vi "Acquire fr Multiple Cameras.vi"() -> (0 "error out":errorcluster)   [LabVIEW 2022 SP3]
uses:
  Anemometry Sub Vis/Globals/Meas_global.vi
  Camera Server/Globals/CamServer global.vi
panel:
  out "element":path
  out "Name 4":string
  out "Image 4":T1(plugin-control)
  out "Name 3":string
  out "Image 3":T1(plugin-control)
  out "Name 2":string
  out "Image 2":T1(plugin-control)
  out "Name 1":string
  out "Image 1":T1(plugin-control)
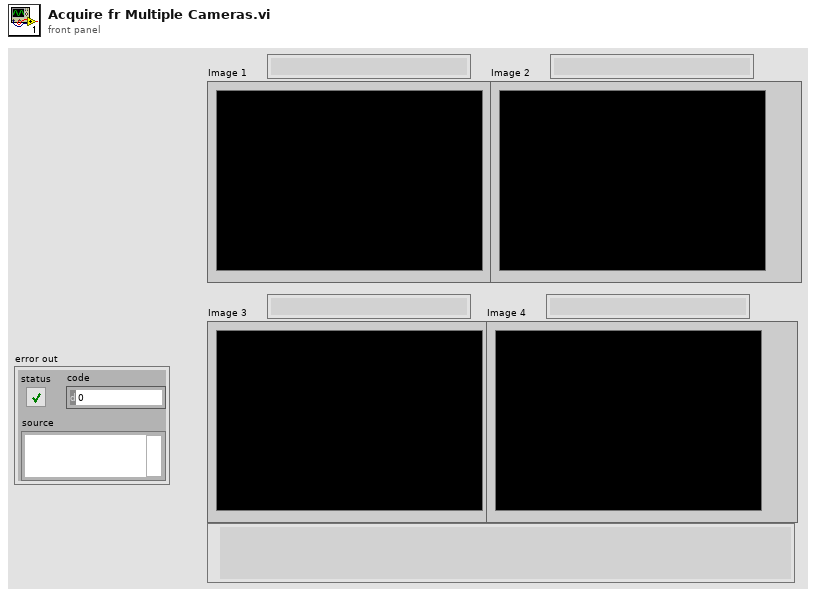
[diagram p1: front panel]
types:
  T1 = typedef "IMAQ Image.ctl" = refnum<image>
  T2 = typedef "Camera enum.ctl" = string
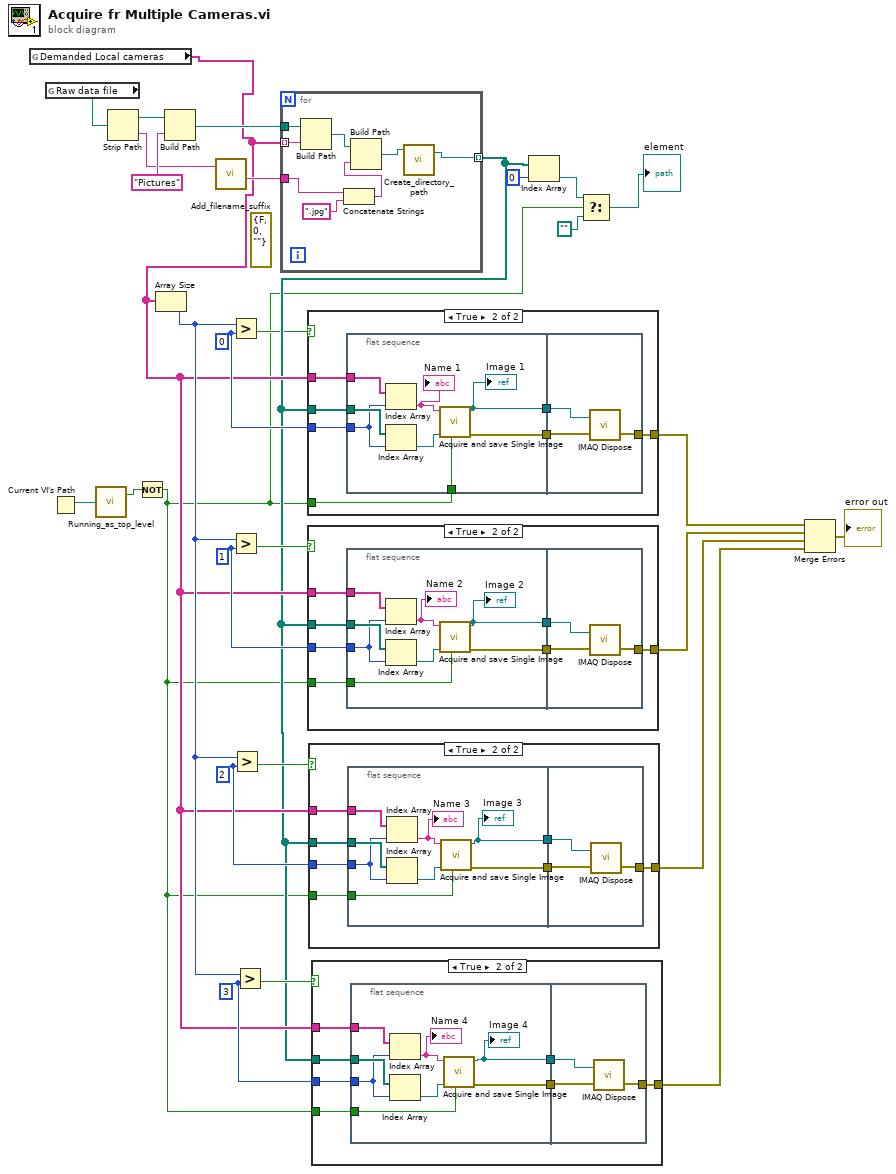
[diagram p0: block diagram]
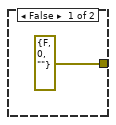
[diagram p2: hidden frame]
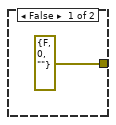
[diagram p3: hidden frame]
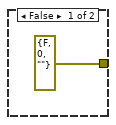
[diagram p4: hidden frame]
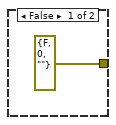
[diagram p5: hidden frame]
diagram:
  w14 = 3 ("y")
  w15 = 2 ("y")
  w16 = 1 ("y")
  w17 = 0 ("y")
  (unwired) errorcluster {"status"=FALSE, "code"=0, "source"=""} ("error IO")
  n1 = global read "CamServer global.vi" "Demanded Local cameras"() -> (w10:T2[])
  n2 = global read "Meas_global.vi" "Raw data file"() -> (w25:path)
  n3 = Current VI's Path() -> (path=w9:path)
  n4 = call "Running_as_top_level.vi"("Vi path name"=w9) -> ("Top Level"=w8:bool)  [unwired: 1 out]
  n5 = Strip Path(path=w25) -> (stripped path=w27:path, name=w24:string)
  n6 = Not(x=w8) -> (.not. x?=w1:bool)
  n7 = Array Size(array=w10) -> (size(s)=w18:i32)
  n8 = Build Path(base path=w27, name or relative path="Pictures") -> (appended path=w28:path)
  n9 = call "Add_filename_suffix.vi"("Filename"=w24) -> ("Base name"=w29:string)  [unwired: 1 in, 3 out]
  n10 = Greater?(x=w18, y=w17) -> (0:w5:bool)
  n11 = Greater?(x=w18, y=w16) -> (0:w21:bool)
  n12 = Greater?(x=w18, y=w15) -> (0:w20:bool)
  n13 = Greater?(x=w18, y=w14) -> (0:w19:bool)
  n14 = for {
    tunnel: w28 -> [w37]
    tunnel: w10 -> [w32] mode=indexing
    tunnel: w29 -> [w33]
    tunnel: [w30] -> w7 mode=indexing
    n15 = Build Path(base path=w37, name or relative path=w32) -> (appended path=w36:path)
    n16 = Concatenate Strings(w33, ".jpg" ("string")) -> (w34:string)
    n17 = Build Path(base path=w36, name or relative path=w34) -> (appended path=w31:path)
    n18 = call "Create_directory_path.vi"("Path name"=w31) -> ("Path name Out"=w30:path)  [unwired: 2 in, 1 out]
  }
  n19 = case shown="True" w5 {
    tunnel: w10 -> [_ w45]
    tunnel: w7 -> [_ w44]
    tunnel: [errorcluster {"status"=FALSE, "code"=0, "source"=""} ("error out") w43] -> w23
    tunnel: w17 -> [_ w40]
    tunnel: w1 -> [_ w39]
    frame False {
    }
    frame True {
      n20 = flat-sequence {
        tunnel: w45 -> [w53]
        tunnel: w44 -> [w52]
        tunnel: [w50] -> w42
        tunnel: [w49] -> w41
        tunnel: w40 -> [w48]
        tunnel: w39 -> [w46]
        tunnel: [w55] -> w43
        tunnel: w42 -> [w56]
        tunnel: w41 -> [w54]
        frame #0 {
          n21 = Index Array(array=w53, index=w48) -> (element=w47:T2)
          "Name 1" <- w47
          n22 = Index Array(array=w52, index=w48) -> (element=w51:path)
          n23 = call "Acquire and save Single Image.vi"("Save image?"=w46, "File Path"=w51, "Camera Name"=w47) -> ("error out"=w50:errorcluster, "Image"=w49:T1)  [unwired: 4 in]
          "Image 1" <- w49
        }
        frame #1 {
          n24 = call "IMAQ Dispose"("Image"=w54, "error in (no error)"=w56) -> ("error out"=w55:errorcluster)  [unwired: 4 in]
        }
      }
    }
  }
  n25 = case shown="True" w21 {
    tunnel: w10 -> [_ w64]
    tunnel: w7 -> [_ w63]
    tunnel: [errorcluster {"status"=FALSE, "code"=0, "source"=""} ("error out") w62] -> w13
    tunnel: w16 -> [_ w59]
    tunnel: w1 -> [_ w58]
    frame False {
    }
    frame True {
      n26 = flat-sequence {
        tunnel: w64 -> [w72]
        tunnel: w63 -> [w71]
        tunnel: [w69] -> w61
        tunnel: [w67] -> w60
        tunnel: w59 -> [w68]
        tunnel: w58 -> [w65]
        tunnel: [w74] -> w62
        tunnel: w61 -> [w75]
        tunnel: w60 -> [w73]
        frame #0 {
          n27 = Index Array(array=w72, index=w68) -> (element=w66:T2)
          "Name 2" <- w66
          n28 = Index Array(array=w71, index=w68) -> (element=w70:path)
          n29 = call "Acquire and save Single Image.vi"("Save image?"=w65, "File Path"=w70, "Camera Name"=w66) -> ("error out"=w69:errorcluster, "Image"=w67:T1)  [unwired: 4 in]
          "Image 2" <- w67
        }
        frame #1 {
          n30 = call "IMAQ Dispose"("Image"=w73, "error in (no error)"=w75) -> ("error out"=w74:errorcluster)  [unwired: 4 in]
        }
      }
    }
  }
  n31 = case shown="True" w20 {
    tunnel: w10 -> [_ w83]
    tunnel: w7 -> [_ w82]
    tunnel: [errorcluster {"status"=FALSE, "code"=0, "source"=""} ("error out") w81] -> w12
    tunnel: w15 -> [_ w78]
    tunnel: w1 -> [_ w77]
    frame False {
    }
    frame True {
      n32 = flat-sequence {
        tunnel: w83 -> [w91]
        tunnel: w82 -> [w90]
        tunnel: [w88] -> w80
        tunnel: [w86] -> w79
        tunnel: w78 -> [w87]
        tunnel: w77 -> [w84]
        tunnel: [w93] -> w81
        tunnel: w80 -> [w94]
        tunnel: w79 -> [w92]
        frame #0 {
          n33 = Index Array(array=w91, index=w87) -> (element=w85:T2)
          "Name 3" <- w85
          n34 = Index Array(array=w90, index=w87) -> (element=w89:path)
          n35 = call "Acquire and save Single Image.vi"("Save image?"=w84, "File Path"=w89, "Camera Name"=w85) -> ("error out"=w88:errorcluster, "Image"=w86:T1)  [unwired: 4 in]
          "Image 3" <- w86
        }
        frame #1 {
          n36 = call "IMAQ Dispose"("Image"=w92, "error in (no error)"=w94) -> ("error out"=w93:errorcluster)  [unwired: 4 in]
        }
      }
    }
  }
  n37 = case shown="True" w19 {
    tunnel: w10 -> [_ w102]
    tunnel: w7 -> [_ w101]
    tunnel: [errorcluster {"status"=FALSE, "code"=0, "source"=""} ("error out") w100] -> w11
    tunnel: w14 -> [_ w97]
    tunnel: w1 -> [_ w96]
    frame False {
    }
    frame True {
      n38 = flat-sequence {
        tunnel: w102 -> [w110]
        tunnel: w101 -> [w109]
        tunnel: [w107] -> w99
        tunnel: [w105] -> w98
        tunnel: w97 -> [w106]
        tunnel: w96 -> [w103]
        tunnel: [w112] -> w100
        tunnel: w99 -> [w113]
        tunnel: w98 -> [w111]
        frame #0 {
          n39 = Index Array(array=w110, index=w106) -> (element=w104:T2)
          "Name 4" <- w104
          n40 = Index Array(array=w109, index=w106) -> (element=w108:path)
          n41 = call "Acquire and save Single Image.vi"("Save image?"=w103, "File Path"=w108, "Camera Name"=w104) -> ("error out"=w107:errorcluster, "Image"=w105:T1)  [unwired: 4 in]
          "Image 4" <- w105
        }
        frame #1 {
          n42 = call "IMAQ Dispose"("Image"=w111, "error in (no error)"=w113) -> ("error out"=w112:errorcluster)  [unwired: 4 in]
        }
      }
    }
  }
  n43 = Index Array(array=w7, index=0) -> (element=w4:path)
  n44 = Select(t=w4, s=w1, f=path "") -> (s? t:f=→"element":path)
  n45 = Merge Errors(w23, w13, w12, w11) -> (→"error out":errorcluster)
